vi "buildApp.vi"(8 "error in (no error)":errorcluster) -> (0 "error out":errorcluster)   [LabVIEW 2018]
doc: "Build the application."
uses:
  <vilib>/AppBuilder/AB_API_Simple/Build (path).vi
  <vilib>/AppBuilder/AB_API_Simple/NI_App_Builder_API.lvlib
panel:
  # "Building the application..please wait."
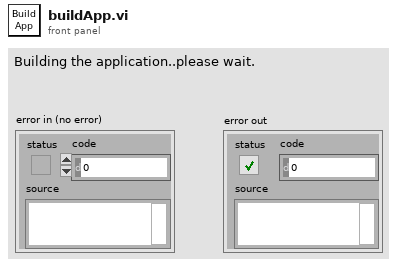
[diagram p1: front panel]
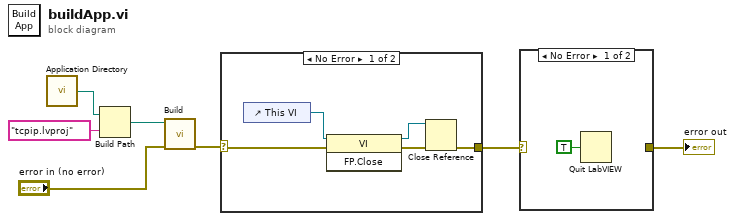
[diagram p0: block diagram]
diagram:
  n1 = call <vilib>:"Application Directory.vi"() -> ("Application Directory"=w7:path)
  n2 = Build Path(base path=w7, name or relative path="tcpip.lvproj") -> (appended path=w5:path)
  n3 = call-poly <vilib>:"Build.vi"("error in (no error)"="error in (no error)", "Path to project"=w5) -> ("error out"=w3:errorcluster)  [unwired: 8 in, 1 out]
  n4 = case shown="No Error" w3 {
    selector: w3 -> [w11 w13]
    tunnel: [w8 w13] -> w2
    frame No Error {
      n5 = control-ref of="This VI"() -> (w12:refnum<vi>)
      n6 = invoke class="VI" method="FP.Close"(reference=w12, error in=w11) -> (reference out=w9:refnum<vi>, error out=w10:errorcluster)  [unwired: 1 in, 1 out]
      n7 = Close Reference(reference=w9, error in (no error)=w10) -> (error out=w8:errorcluster)
    }
    frame Error {
    }
  }
  n8 = case shown="No Error" w2 {
    selector: w2 -> [_ w15]
    tunnel: [_ w15] -> w1
    frame No Error {
      n9 = Quit LabVIEW(quit? (T)=TRUE) -> ()
    }
    frame Error {
    }
  }
  "error out" <- w1
